vi "Convert UTF-8 to LV Text.vi"(7 "UTF-8 Text":string, 9 "error in":errorcluster) -> (8 "LV Text":string, 10 "error out":errorcluster)   [LabVIEW 2017]
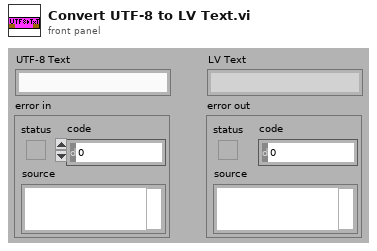
[diagram p1: front panel]
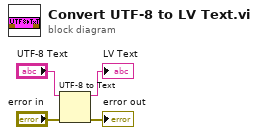
[diagram p0: block diagram]
diagram:
  n1 = UTF-8 to Text(8:"error in", 11:"UTF-8 Text") -> (0:→"error out":errorcluster, 3:→"LV Text":string)  [unwired: 1 in]
